vi "getAllDevices.vi"(8 "error in (no error)":errorcluster, 11 "DeviceArray.lvclass in":refnum<class "DeviceArray.lvclass">) -> (0 "error out":errorcluster, 2 "deviceArray":refnum<class "device.lvclass">[](array[class]), 3 "DeviceArray.lvclass out":refnum<class "DeviceArray.lvclass">)   [LabVIEW 2009, in "Tools.lvlib" / "DatabaseHelpers.lvlib" / "DeviceArray.lvclass"]
uses:
  DeviceArray.lvclass
  device/device.lvclass
  DeviceArray.lvclass/DeviceArray.ctl
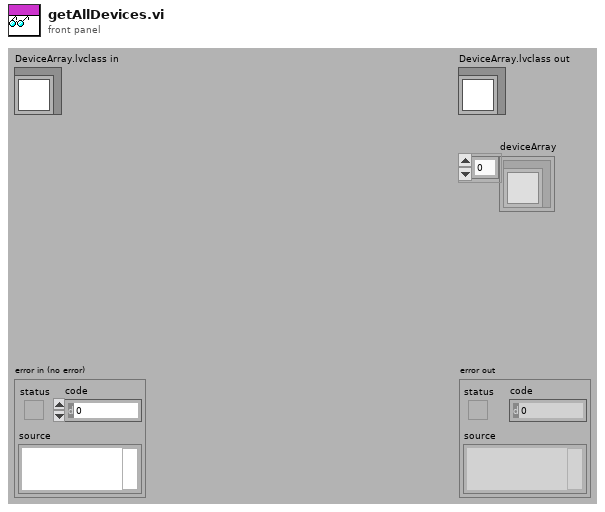
[diagram p1: front panel]
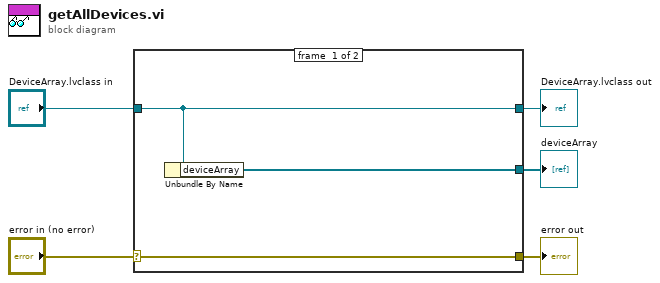
[diagram p0: block diagram]
diagram:
  n1 = case shown="No Error" "error in (no error)" {
    selector: "error in (no error)" -> [w8 w9]
    tunnel: [w8 w9] -> w4
    tunnel: [w7 w10] -> w2
    tunnel: "DeviceArray.lvclass in" -> [w7 w10]
    tunnel: [w6 _] -> w1
    frame #0 {
      n2 = Unbundle By Name(w7) -> ("deviceArray"=w6:refnum<class "device.lvclass">[])
    }
    frame #1 {
    }
  }
  "error out" <- w4
  "DeviceArray.lvclass out" <- w2
  "deviceArray" <- w1
